vi "Input_to_Dash.vi"(1 "error in (no error)":errorcluster, 2 "Select Type":string(combo)="String", 3 "Dashboard Value":string, 4 "Input - Array":void[](array[numeric]), 5 "Input - Cluster":cluster{}, 6 "Input - Int":dbl, 7 "Input - String":string) -> ()   [LabVIEW 2016]
uses:
  <vilib>/Rock Robotics/Network Tables/NT Write Numeric Array.vi
panel:
  out "error out":errorcluster
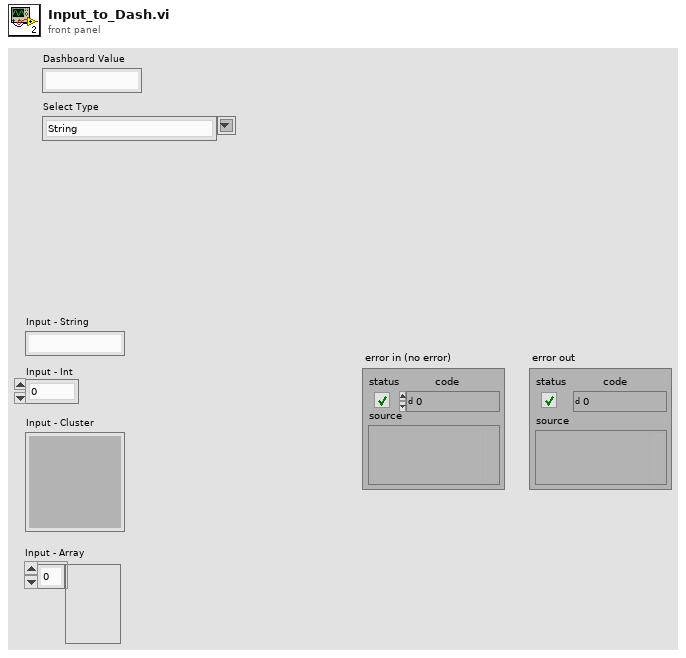
[diagram p1: front panel]
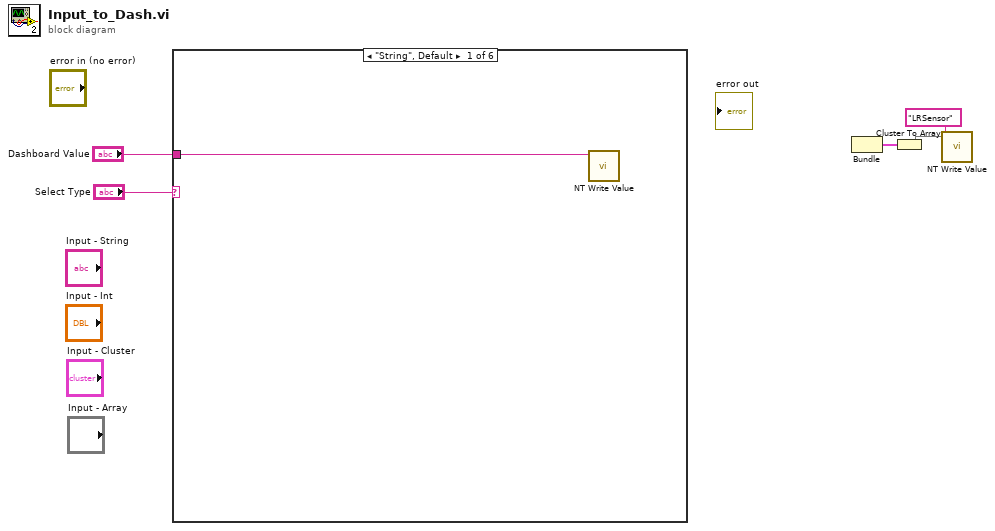
[diagram p0: block diagram]
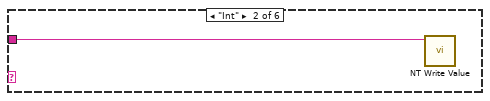
[diagram p2: hidden frame]
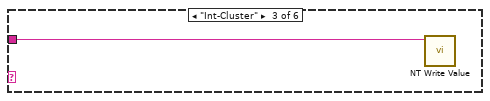
[diagram p3: hidden frame]
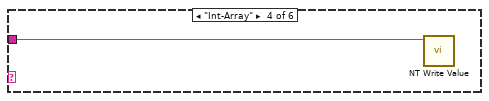
[diagram p4: hidden frame]
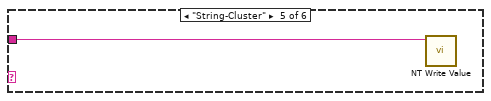
[diagram p5: hidden frame]
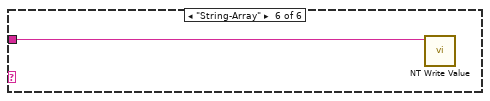
[diagram p6: hidden frame]
diagram:
  n1 = case shown="\"String\", Default" "Select Type" {
    tunnel: "Dashboard Value" -> [w6 w7 w8 w9 w10 w11]
    frame "String", Default {
      n2 = call-poly <vilib>:"NT Write Value.vi"("Name"=w6) -> ()  [unwired: 10 in, 1 out]
    }
    frame "Int" {
      n3 = call-poly <vilib>:"NT Write Value.vi"("Name"=w7) -> ()  [unwired: 10 in, 1 out]
    }
    frame "Int-Cluster" {
      n4 = call-poly <vilib>:"NT Write Value.vi"("Name"=w8) -> ()  [unwired: 10 in, 1 out]
    }
    frame "Int-Array" {
      n5 = call-poly <vilib>:"NT Write Value.vi"("Name"=w9) -> ()  [unwired: 10 in, 1 out]
    }
    frame "String-Cluster" {
      n6 = call-poly <vilib>:"NT Write Value.vi"("Name"=w10) -> ()  [unwired: 10 in, 1 out]
    }
    frame "String-Array" {
      n7 = call-poly <vilib>:"NT Write Value.vi"("Name"=w11) -> ()  [unwired: 10 in, 1 out]
    }
  }
  n8 = Bundle() -> (w3:cluster{void, void})  [unwired: 3 in]
  n9 = Cluster To Array(cluster=w3) -> (array=w2:void[])
  n10 = call-poly <vilib>:"NT Write Value.vi"("Numeric Array"=w2, "Name"="LRSensor") -> ()  [unwired: 9 in, 1 out]
